vi "Write Template Paths.vi"(8 "error in (no error)":errorcluster, 10 "Template Paths":path[](array[path]), 11 "CS++MessageMakerMain in":refnum<class "CS++MessageMakerMain.lvclass">) -> (0 "error out":errorcluster, 3 "CS++MessageMakerMain out":refnum<class "CS++MessageMakerMain.lvclass">)   [LabVIEW 2016, in "CS++MessageMakerMain.lvlib" / "CS++MessageMakerMain.lvclass"]
uses:
  CS++MessageMakerMain.lvclass
  CS++MessageMakerMain.lvclass/CS++MessageMakerMain.ctl
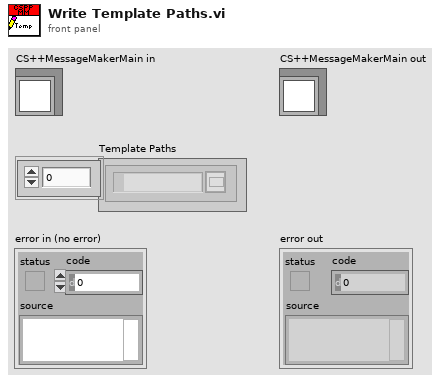
[diagram p1: front panel]
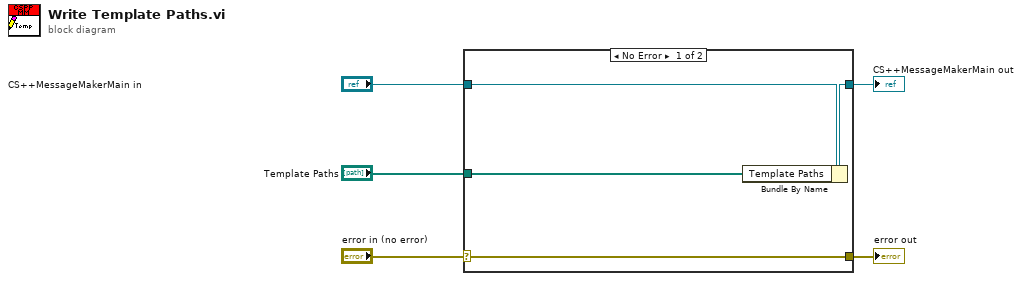
[diagram p0: block diagram]
diagram:
  n1 = case shown="No Error" "error in (no error)" {
    selector: "error in (no error)" -> [w9 w10]
    tunnel: [w9 w10] -> w4
    tunnel: [w7 w11] -> w2
    tunnel: "CS++MessageMakerMain in" -> [w8 w11]
    tunnel: "Template Paths" -> [w6 _]
    frame No Error {
      n2 = Bundle By Name(cluster=w8, "Template Paths"=w6) -> (w7:refnum<class "CS++MessageMakerMain.lvclass">)
    }
    frame Error {
    }
  }
  "error out" <- w4
  "CS++MessageMakerMain out" <- w2
